vi "Stop Core.vi"(10 "final error code":i32, 11 "ZWO_ASI in":refnum<class "ZWO_ASI.lvclass">) -> (3 "ZWO_ASI out":refnum<class "ZWO_ASI.lvclass">)   [LabVIEW 2023, in "ZWO_ASI.lvlib" / "ZWO_ASI.lvclass"]
doc: "(<B>Filename</B>: Actor Framework.lvlib:Actor.lvclass:Stop Core.vi)\n\nDefines what the actor does before it stops. Use the <B>final error code</B> input to determine whether the actor shut down in response to an error.\n\nBy default, this method passes the Stop message along to all auto-stop nested actors. A descendant class may override this method to define additional behavior, such as shutting down any processes the actor initiated in its override of the Actor Core method."
uses:
  ZWO_ASI.lvclass
  <vilib>/ActorFramework/Actor/Actor.lvclass
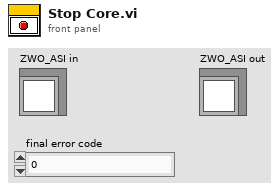
[diagram p1: front panel]
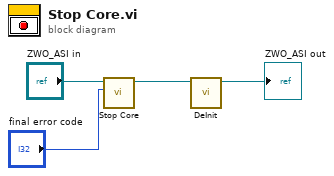
[diagram p0: block diagram]
diagram:
  n1 = call-parent "Stop Core.vi"("final error code"="final error code", "Actor in"="ZWO_ASI in") -> ("Actor out"=w2:refnum<class "ZWO_ASI.lvclass">)  [unwired: 9 in]
  n2 = call-dynamic "DeInit.vi"("ZWO_ASI in"=w2) -> ("ZWO_ASI out"=→"ZWO_ASI out":refnum<class "ZWO_ASI.lvclass">)  [unwired: 9 in, 1 out]
